vi "Create Stock Requests.vi"(8 "error in":errorcluster, 10 "Method Name":string, 11 "Method":T2) -> (0 "error out":errorcluster)   [LabVIEW 2011]
uses:
  Method.ctl
  RequestKeys.ctl
  Folders.ctl
  Design Server.lvlib
panel:
  in  "Request Keys":T1
  in  "Default Values":string[](array[string])=["METHOD", "Stock Design", "", "", "", "PROJECTTITLE", "", "", ""]
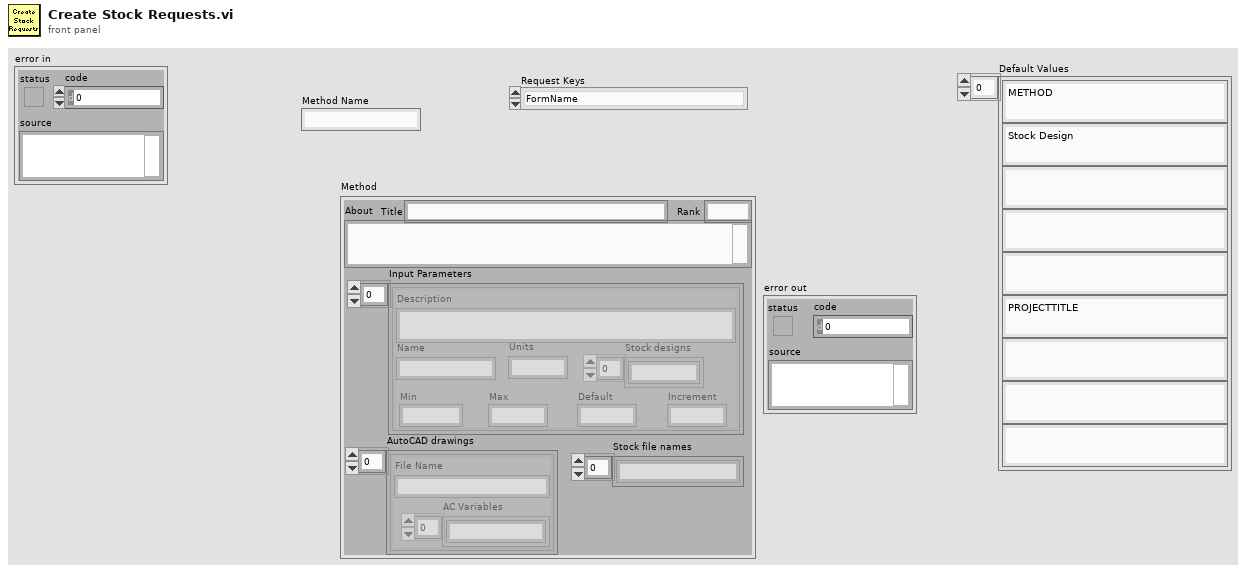
[diagram p1: front panel]
types:
  T1 = typedef "Design Server.lvlib/RequestKeys.ctl" = enum16{"FormName", "Name", "Email", "Organization", "Country", "ProjectTitle", "ProjectCity", "ProjectState", "ProjectNotes"}
  T2 = typedef "Method.ctl" = cluster{"Title":string, "Rank":string, "About":string, "Input Parameters":cluster{"Description":string, "Name":string, "Min":string, "Max":string, "Default":string, "Units":string, "Increment":string, "Stock designs":string[]}[], "AutoCAD drawings":cluster{"File Name":string, "AC Variables":string[]}[], "Stock file names":string[]}
  T3 = typedef "Design Server.lvlib/Folders.ctl" = enum16{"MathcadMethods", "RequestedDesigns", "CompletedDesigns", "MathcadCode", "CollabnetSVN.exe"}
  T4 = cluster{"Description":string, "Name":string, "Min":string, "Max":string, "Default":string, "Units":string, "Increment":string, "Stock designs":string[]}[]
  T5 = enum16{"open", "replace", "create", "open or create", "replace or create", "replace or create with confirmation"}
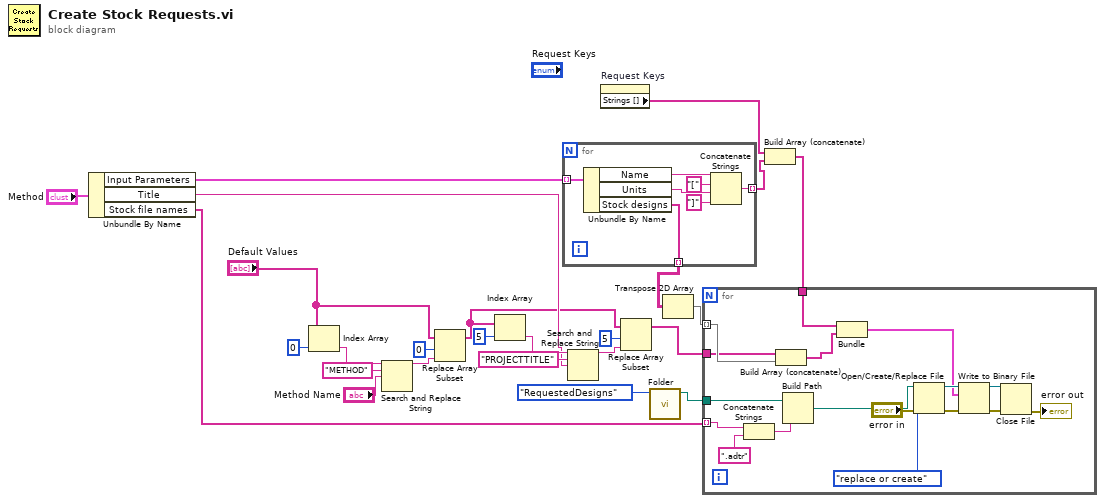
[diagram p0: block diagram]
diagram:
  n1 = Unbundle By Name("Method") -> ("Input Parameters"=w23:T4, "Title"=w4:string, "Stock file names"=w10:string[])
  n2 = Index Array(array="Default Values", index=0) -> (element=w16:string)
  n3 = Search and Replace String(input string=w16, search string="METHOD", replace string="Method Name") -> (result string=w11:string)  [unwired: 5 in, 3 out]
  n4 = Replace Array Subset(array="Default Values", new element=w11, index=0) -> (w3:string[])
  n5 = Index Array(array=w3, index=5) -> (element=w6:string)
  n6 = for {
    tunnel: w23 -> [w32] mode=indexing
    tunnel: [w27] -> w22 mode=indexing
    tunnel: [w26] -> w21 mode=indexing
    n7 = Unbundle By Name(w32) -> ("Name"=w31:string, "Units"=w30:string, "Stock designs"=w26:string[])
    n8 = Concatenate Strings(w31, "[" ("string"), w30, "]" ("string")) -> (w27:string)
  }
  n9 = Search and Replace String(input string=w6, search string="PROJECTTITLE", replace string=w4) -> (result string=w9:string)  [unwired: 5 in, 3 out]
  n10 = property on="Request Keys" class="Enum (strict)"() -> ("Strings []"=w1:string[])  [unwired: 2 in, 2 out]
  n11 = Replace Array Subset(array=w3, new element=w9, index=5) -> (w2:string[])
  n12 = call "Folder.vi"("Folders"=Folders."RequestedDesigns") -> ("FolderPath"=w18:path)  [unwired: 8 in, 2 out]
  n13 = Transpose 2D Array(2D array=w21) -> (transposed array=w20:string[][])
  n14 = Build Array (concatenate)(w1, w22) -> (w19:string[])
  n15 = for {
    tunnel: w20 -> [w49] mode=indexing
    tunnel: w19 -> [w48]
    tunnel: w10 -> [w41] mode=indexing
    tunnel: w18 -> [w43]
    tunnel: w2 -> [w33]
    n16 = Concatenate Strings(w41, ".adtr") -> (w40:string)
    n17 = Build Array (concatenate)(w33, w49) -> (w47:string[])
    n18 = Build Path(base path=w43, name or relative path=w40) -> (appended path=w39:path)
    n19 = Bundle(w48, w47) -> (w37:cluster{string[], string[]})  [unwired: 1 in]
    n20 = Open/Create/Replace File(file path (use dialog)=w39, error in="error in", operation (0:open)=T5."replace or create") -> (refnum out=w38:refnum<file>, error out=w46:errorcluster)  [unwired: 3 in, 1 out]
    n21 = Write to Binary File(file (use dialog)=w38, data=w37, error in=w46) -> (refnum out=w44:refnum<file>, error out=w45:errorcluster)  [unwired: 3 in, 1 out]
    n22 = Close File(refnum=w44, error in=w45) -> (error out=→"error out":errorcluster)  [unwired: 1 out]
  }
